vi "Get All Data.vi"(0 "I2C Ref In":T1={"myRIO Reference"={"myRIO Model"=enum."Unknown", "myRIO Hardware Reference"={"Generic FPGA Reference"=refnum, "Allow multiple opens"=FALSE}}, "I2C Channels Enum"=enum."Not Connected", "I2C Configuration"={"I2C Transfer Rate"=enum."Fast mode (400 kbps)"}}, 5 "Device Address":T9=104 items=["0x68"=104, "0x69"=105], 11 "error in (no error)":errorcluster) -> (4 "I2C Ref Out":T1={"myRIO Reference"={"myRIO Model"=enum."Unknown", "myRIO Hardware Reference"={"Generic FPGA Reference"=refnum, "Allow multiple opens"=FALSE}}, "I2C Channels Enum"=enum."Not Connected", "I2C Configuration"={"I2C Transfer Rate"=enum."Fast mode (400 kbps)"}}, 6 "Accel Data":T10, 8 "Temperature (°C)":dbl, 10 "Gyro Data":T10, 15 "error out":errorcluster)   [LabVIEW 2017]
uses:
  DeviceAddresses.ctl
  <vilib>/myRIO/Instrument Drivers/Onboard IO/I2C/typedefs/I2C Reference.ctl
  <vilib>/myRIO/Common/Instrument Driver Framework/Utilities/typedefs/myRIO Generic Hardware Reference.ctl
  <vilib>/myRIO/Common/Instrument Driver Framework/Utilities/typedefs/Hardware Version Enum.ctl
  <vilib>/myRIO/Common/Instrument Driver Framework/Utilities/typedefs/myRIO v1.0 Reference.ctl
  <vilib>/myRIO/Common/Instrument Driver Framework/Utilities/typedefs/Generic FPGA Reference.ctl
  <vilib>/myRIO/Common/Instrument Driver Framework/myRIO v1.0/I2C/typedefs/I2C Channels Enum.ctl
  <vilib>/myRIO/Instrument Drivers/Onboard IO/I2C/typedefs/I2C Configuration.ctl
  <vilib>/myRIO/Instrument Drivers/Onboard IO/I2C/typedefs/I2C Transfer Rate.ctl
  RegisterAddresses.ctl
  <vilib>/Utility/error.llb/Error Cluster From Error Code.vi
  <vilib>/myRIO/Common/Instrument Driver Framework/myRIO v1.0/I2C/vis/myRIO v1.0 Write I2C.vi
  <vilib>/myRIO/Common/Instrument Driver Framework/myRIO v1.0/I2C/vis/myRIO v1.0 Read I2C.vi
  <vilib>/myRIO/Instrument Drivers/Onboard IO/I2C/I2C.lvlib
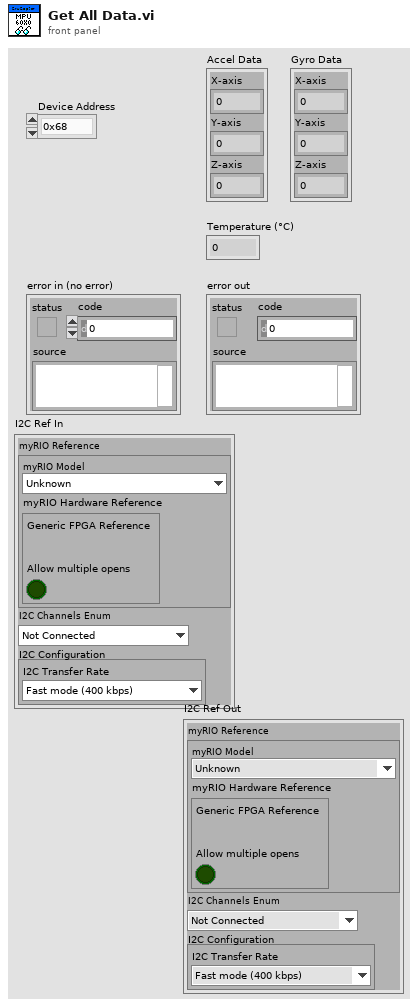
[diagram p1: front panel]
types:
  T1 = typedef "I2C.lvlib/I2C Reference.ctl" = cluster{"myRIO Reference":T2, "I2C Channels Enum":T6, "I2C Configuration":T7}
  T2 = typedef "myRIO Generic Hardware Reference.ctl" = cluster{"myRIO Model":T3, "myRIO Hardware Reference":T4}
  T3 = typedef "Hardware Version Enum.ctl" = enum16{"Unknown", "myRIO-1900", "myRIO-1950", "roboRIO", "NI ELVIS RIO CM"}
  T4 = typedef "myRIO v1.0 Reference.ctl" = cluster{"Generic FPGA Reference":T5, "Allow multiple opens":bool}
  T5 = typedef "Generic FPGA Reference.ctl" = refnum<k20>
  T6 = typedef "I2C Channels Enum.ctl" = enum16{"Not Connected", "A/I2C", "B/I2C", "I2C/I2C"}
  T7 = typedef "I2C.lvlib/I2C Configuration.ctl" = cluster{"I2C Transfer Rate":T8}
  T8 = typedef "I2C.lvlib/I2C Transfer Rate.ctl" = enum16{"Standard mode (100 kbps)", "Fast mode (400 kbps)"}
  T9 = typedef "DeviceAddresses.ctl" = u8
  T10 = cluster{"X-axis":i16, "Y-axis":i16, "Z-axis":i16}
  T11 = typedef "RegisterAddresses.ctl" = u16
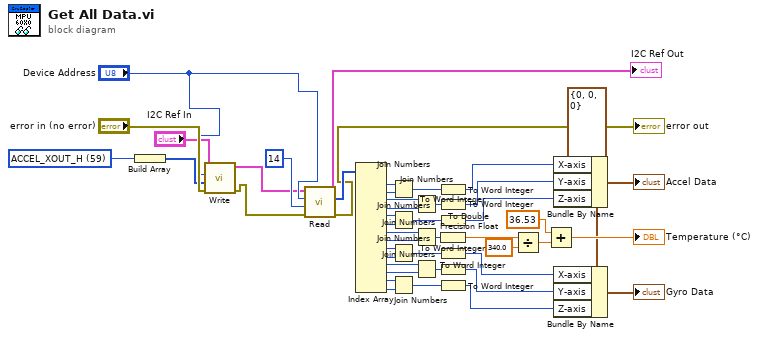
[diagram p0: block diagram]
diagram:
  w15 = T10 {"X-axis"=0, "Y-axis"=0, "Z-axis"=0} ("input cluster")
  w46 = T11 59 items=["SELF_TEST_X"=13, "SELF_TEST_Y"=14, "SELF_TEST_Z"=15, "SELF_TEST_A"=16, "SMPLRT_DIV"=25, "CONFIG"=26, "GYRO_CONFIG"=27, "ACCEL_CONFIG"=28, "MOT_THR"=31, "FIFO_EN"=35, "I2C_MST_CTRL"=36, "I2C_SLV0_ADDR"=37, "I2C_SLV0_REG"=38, "I2C_SLV0_CTRL"=39, "I2C_SLV1_ADDR"=40, "I2C_SLV1_REG"=41, "I2C_SLV1_CTRL"=42, "I2C_SLV2_ADDR"=43, "I2C_SLV2_REG"=44, "I2C_SLV2_CTRL"=45, "I2C_SLV3_ADDR"=46, "I2C_SLV3_REG"=47, "I2C_SLV3_CTRL"=48, "I2C_SLV4_ADDR"=49, "I2C_SLV4_REG"=50, "I2C_SLV4_DO"=51, "I2C_SLV4_CTRL"=52, "I2C_SLV4_DI"=53, "I2C_MST_STATUS"=54, "INT_PIN_CFG"=55, "INT_ENABLE"=56, "INT_STATUS"=58, "ACCEL_XOUT_H"=59, "ACCEL_XOUT_L"=60, "ACCEL_YOUT_H"=61, "ACCEL_YOUT_L"=62, "ACCEL_ZOUT_H"=63, "ACCEL_ZOUT_L"=64, "TEMP_OUT_H"=65, "TEMP_OUT_L"=66, "GYRO_XOUT_H"=67, "GYRO_XOUT_L"=68, "GYRO_YOUT_H"=69, "GYRO_YOUT_L"=70, "GYRO_ZOUT_H"=71, "GYRO_ZOUT_L"=72, "EXT_SENS_DATA_00"=73, "EXT_SENS_DATA_01"=74, "EXT_SENS_DATA_02"=75, "EXT_SENS_DATA_03"=76, "EXT_SENS_DATA_04"=77, "EXT_SENS_DATA_05"=78, "EXT_SENS_DATA_06"=79, "EXT_SENS_DATA_07"=80, "EXT_SENS_DATA_08"=81, "EXT_SENS_DATA_09"=82, "EXT_SENS_DATA_10"=83, "EXT_SENS_DATA_11"=84, "EXT_SENS_DATA_12"=85, "EXT_SENS_DATA_13"=86, "EXT_SENS_DATA_14"=87, "EXT_SENS_DATA_15"=88, "EXT_SENS_DATA_16"=89, "EXT_SENS_DATA_17"=90, "EXT_SENS_DATA_18"=91, "EXT_SENS_DATA_19"=92, "EXT_SENS_DATA_20"=93, "EXT_SENS_DATA_21"=94, "EXT_SENS_DATA_22"=95, "EXT_SENS_DATA_23"=96, "I2C_SLV0_DO"=99, "I2C_SLV1_DO"=100, "I2C_SLV2_DO"=101, "I2C_SLV3_DO"=102, "I2C_MST_DELAY_CTRL"=103, "SIGNAL_PATH_RESET"=104, "MOT_DETECT_CTRL"=105, "USER_CTRL"=106, "PWR_MGMT_1"=107, "PWR_MGMT_2"=108, "FIFO_COUNTH"=114, "FIFO_COUNTL"=115, "FIFO_R_W"=116, "WHO_AM_I"=117] ("Register Addresses")
  n1 = Build Array(w46) -> (w9:T11[])
  n2 = call <vilib>:"Write.vi"("error in (no error)"="error in (no error)", "Bytes to Write"=w9, "Slave Address (7-bit)"="Device Address", "I2C Ref In"="I2C Ref In") -> ("error out"=w4:errorcluster, "I2C Ref Out"=w5:T1)  [unwired: 6 in]
  n3 = call <vilib>:"Read.vi"("error in (no error)"=w4, "Byte Count"=u8 14 ("Bytes To Read"), "Slave Address (7-bit)"="Device Address", "I2C Ref In"=w5) -> ("error out"=→"error out":errorcluster, "Bytes Read"=w3:u8[], "I2C Ref Out"=→"I2C Ref Out":T1)  [unwired: 4 in]
  n4 = Index Array(array=w3) -> (element #1=w45:u8, element #2=w44:u8, element #3=w43:u8, element #4=w42:u8, element #5=w41:u8, element #6=w40:u8, element #7=w39:u8, element #8=w38:u8, element #9=w37:u8, element #10=w36:u8, element #11=w35:u8, element #12=w34:u8, element #13=w33:u8, element #14=w32:u8)  [unwired: 14 in]
  n5 = Join Numbers(hi=w45, lo=w44) -> ((hi.lo)=w30:u16)
  n6 = Join Numbers(hi=w41, lo=w40) -> ((hi.lo)=w29:u16)
  n7 = Join Numbers(hi=w37, lo=w36) -> ((hi.lo)=w25:u16)
  n8 = Join Numbers(hi=w33, lo=w32) -> ((hi.lo)=w26:u16)
  n9 = Join Numbers(hi=w43, lo=w42) -> ((hi.lo)=w31:u16)
  n10 = Join Numbers(hi=w39, lo=w38) -> ((hi.lo)=w28:u16)
  n11 = Join Numbers(hi=w35, lo=w34) -> ((hi.lo)=w27:u16)
  n12 = To Word Integer(number=w30) -> (16bit integer=w19:i16)
  n13 = To Word Integer(number=w31) -> (16bit integer=w18:i16)
  n14 = To Word Integer(number=w29) -> (16bit integer=w17:i16)
  n15 = To Double Precision Float(number=w28) -> (double precision float=w24:dbl)
  n16 = To Word Integer(number=w25) -> (16bit integer=w14:i16)
  n17 = To Word Integer(number=w27) -> (16bit integer=w13:i16)
  n18 = To Word Integer(number=w26) -> (16bit integer=w12:i16)
  n19 = Divide(x=w24, y=340.0) -> (x/y=w22:dbl)
  n20 = Add(x=36.53, y=w22) -> (x+y=→"Temperature (°C)":dbl)
  n21 = Bundle By Name(cluster=w15, "X-axis"=w19, "Y-axis"=w18, "Z-axis"=w17) -> (→"Accel Data":T10)
  n22 = Bundle By Name(cluster=w15, "X-axis"=w14, "Y-axis"=w13, "Z-axis"=w12) -> (→"Gyro Data":T10)
